vi "Find File.vi"(8 "error in (no error)":errorcluster, 11 "File Name":string) -> (0 "error out":errorcluster, 3 "Path":path)   [LabVIEW 2019, in "SMO.Control Experiment.lvclass"]
uses:
  SMO.Control Experiment.lvclass
  <vilib>/Utility/error.llb/Error Cluster From Error Code.vi
  <userlib>/_OpenG.lib/string/string.llb/To Proper Case (String)__ogtk.vi
  <vilib>/ErrorRing/Error Ring.xnode
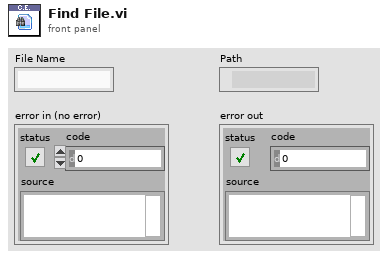
[diagram p1: front panel]
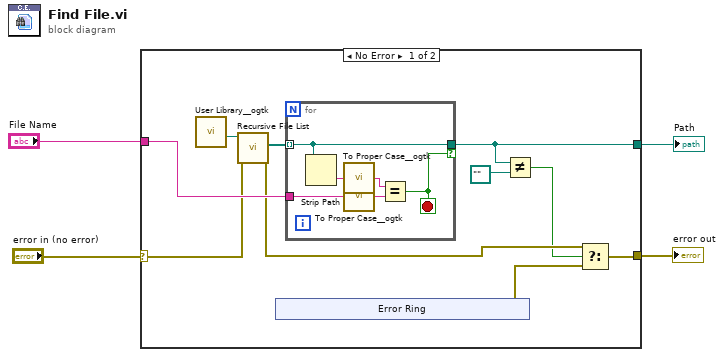
[diagram p0: block diagram]
diagram:
  n1 = case shown="No Error" "error in (no error)" {
    selector: "error in (no error)" -> [w11 w25]
    tunnel: [w6 w25] -> w4
    tunnel: [w9 _] -> w3
    tunnel: "File Name" -> [w14 _]
    frame No Error {
      n2 = call <userlib>:"User Library__ogtk.vi"() -> ("User Library (+ Relative)"=w12:path)  [unwired: 1 in]
      n3 = call <vilib>:"Recursive File List.vi"("error in (no error)"=w11, "Folder Path"=w12) -> ("error out"=w8:errorcluster, "All Files in Dir"=w13:path[])  [unwired: 5 in, 3 out]
      n4 = xnode "Error Ring"() -> ("error out"=w7:errorcluster)
      n5 = for {
        tunnel: w13 -> [w24] mode=indexing
        tunnel: w14 -> [w22]
        tunnel: [w24] -> w9 if=w23
        stop <- w23 stop-if-true
        n6 = Strip Path(path=w24) -> (name=w20:string)  [unwired: 1 out]
        n7 = call-poly <userlib>:"To Proper Case__ogtk.vi"("string"=w20) -> ("proper case string"=w19:string)  [unwired: 4 in]
        n8 = call-poly <userlib>:"To Proper Case__ogtk.vi"("string"=w22) -> ("proper case string"=w21:string)  [unwired: 4 in]
        n9 = Equal?(x=w19, y=w21) -> (x = y?=w23:bool)
      }
      n10 = Not Equal?(x=w9, y=path "") -> (x != y?=w5:bool)
      n11 = Select(t=w8, s=w5, f=w7) -> (s? t:f=w6:errorcluster)
    }
    frame Error {
    }
  }
  "error out" <- w4
  "Path" <- w3
